vi "Generate Minesweeper Drawing Event.vi"(0 "User Event In":refnum<user-event>, 5 "Minesweeper Drawing Operation":T1, 7 "row":i16, 9 "column":i16, 11 "Error In":errorcluster) -> (4 "User Event Out":refnum<user-event>, 15 "Error Out":errorcluster)   [LabVIEW 2011]
uses:
  Minesweeper Drawing Operation Type Def.ctl
  Minesweeper Drawing Event Type Def.ctl
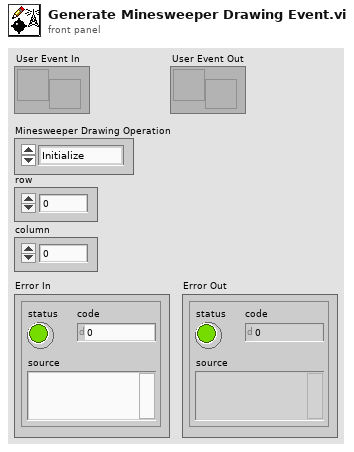
[diagram p1: front panel]
types:
  T1 = typedef "Minesweeper Drawing Operation Type Def.ctl" = enum16{"Initialize", "Uncover", "Flag", "Unflag"}
  T2 = typedef "Minesweeper Drawing Event Type Def.ctl" = cluster{"Minesweeper Drawing Operation":T1, "Operation Index (row, column)":cluster{"x":i16, "y":i16}}
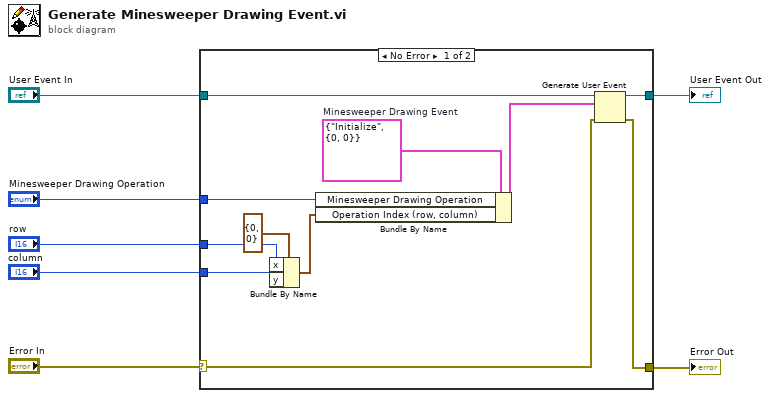
[diagram p0: block diagram]
diagram:
  n1 = case shown="No Error" "Error In" {
    selector: "Error In" -> [w8 w19]
    tunnel: "row" -> [w16 _]
    tunnel: "column" -> [w15 _]
    tunnel: "Minesweeper Drawing Operation" -> [w14 _]
    tunnel: [w12 w19] -> w4
    tunnel: "User Event In" -> [w11 w20]
    tunnel: [w9 w20] -> w2
    frame No Error {
      w18 = T2 {"Minesweeper Drawing Operation"=enum."Initialize", "Operation Index (row, column)"={"x"=0, "y"=0}}  # Minesweeper Drawing Event
      n2 = Bundle By Name(cluster=cluster{"x":i16, "y":i16} {"x"=0, "y"=0} ("Operation Index (row, column)"), "x"=w16, "y"=w15) -> (w17:cluster{"x":i16, "y":i16})
      n3 = Bundle By Name(cluster=w18, "Minesweeper Drawing Operation"=w14, "Operation Index (row, column)"=w17) -> (w10:T2)
      n4 = Generate User Event(user event=w11, event data cluster=w10, error in=w8) -> (user event out=w9:refnum<user-event>, error out=w12:errorcluster)
    }
    frame Error {
    }
  }
  "Error Out" <- w4
  "User Event Out" <- w2
